vi "EnFlo_Inlet_Setpoint_Names.vi"() -> (0 "Sub Names":string[](array[string]))   [LabVIEW 2010]
panel:
  out "Setpoints":dbl[](array[numeric])
  in  "Reload from file":bool
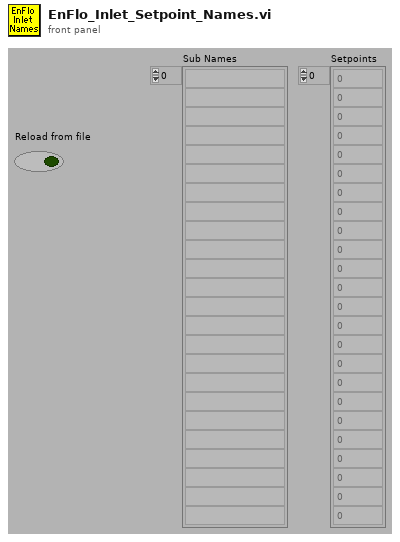
[diagram p1: front panel]
types:
  T1 = typedef "Heater_Setpoint.ctl" = cluster{"Ch Name":string, "Setpoint":dbl}
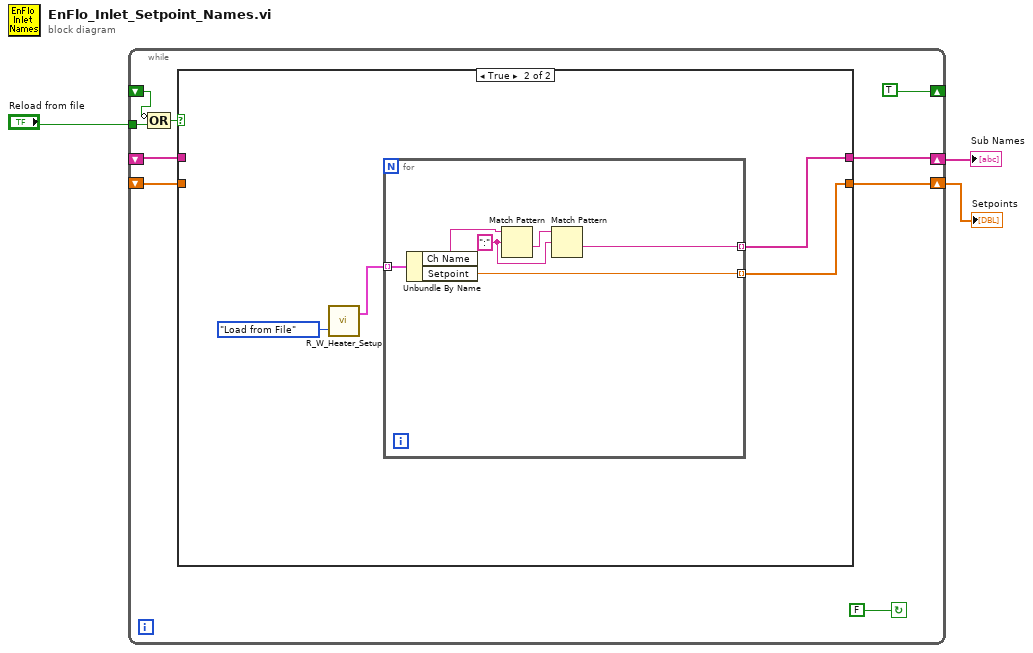
[diagram p0: block diagram]
diagram:
  n1 = while {
    shift-left: _ -> [w7]
    shift-right: [TRUE] -> _
    shift-left: _ -> [w10]
    shift-right: [w12] -> w3
    tunnel: "Reload from file" -> [w8]
    shift-right: [w5] -> w1
    shift-left: _ -> [w4]
    stop <- FALSE continue-if-true
    n2 = Compound Arithmetic op=OR(invert w7, w8) -> (w6:bool)
    n3 = case shown="True" w6 {
      tunnel: [w14 w16] -> w12
      tunnel: w10 -> [w14 _]
      tunnel: [w13 w15] -> w5
      tunnel: w4 -> [w13 _]
      frame False {
      }
      frame True {
        n4 = call "R_W_Heater_Setup.vi"("Mode"=enum16{"Load from File", "Save to File"}."Load from File") -> ("Setpoints Out"=w17:T1[])  [unwired: 1 in, 1 out]
        n5 = for {
          tunnel: w17 -> [w24] mode=indexing
          tunnel: [w20] -> w16 mode=indexing
          tunnel: [w19] -> w15 mode=indexing
          w21 = ":" ("regular expression")
          n6 = Unbundle By Name(w24) -> ("Ch Name"=w23:string, "Setpoint"=w19:dbl)
          n7 = Match Pattern(string=w23, regular expression=w21) -> (after substring=w22:string)  [unwired: 4 out]
          n8 = Match Pattern(string=w22, regular expression=w21) -> (after substring=w20:string)  [unwired: 4 out]
        }
      }
    }
  }
  "Sub Names" <- w3
  "Setpoints" <- w1
